vi "All Rounds.vi"(1 "Hash Function in":refnum<class "NI_SHA-3.lvclass">) -> (0 "Hash Function out":refnum<class "NI_SHA-3.lvclass">)   [LabVIEW 2020, in "NI_SHA-3.lvclass"]
uses:
  <vilib>/security/Message Digest/SHA-3/NI_SHA-3.lvclass
  <vilib>/security/Message Digest/SHA-3/NI_SHA-3.lvclass/NI_SHA-3.ctl
  a6197f31-9067-4d7d-80c5-9a64d9879faa.vi
  a6197f31-9067-4d7d-80c5-9a64d9879faa.vi/a07fe380-13ad-3f96-aad6-c8c87e91e43f.vi
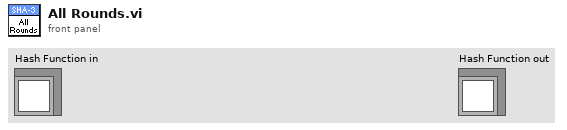
[diagram p1: front panel]
types:
  T1 = typedef "NI_SHA-3.lvclass/state.ctl" = cluster{"A00":T2, "A01":T2, "A02":T2, "A03":T2, "A04":T2, "A05":T2, "A06":T2, "A07":T2, "A08":T2, "A09":T2, "A10":T2, "A11":T2, "A12":T2, "A13":T2, "A14":T2, "A15":T2, "A16":T2, "A17":T2, "A18":T2, "A19":T2, "A20":T2, "A21":T2, "A22":T2, "A23":T2, "A24":T2}
  T2 = typedef "NI_SHA-3.lvclass/state word.ctl" = u64
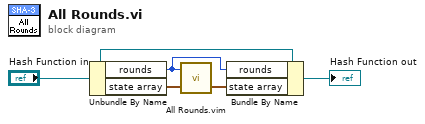
[diagram p0: block diagram]
diagram:
  n1 = Unbundle By Name("Hash Function in") -> ("rounds"=w3:i32, "state array"=w1:T1)
  n2 = call "All Rounds.vim"("state in"=w1, "rounds"=w3) -> ("state out"=w2:T1)  [unwired: 1 in]
  n3 = Bundle By Name(cluster="Hash Function in", "rounds"=w3, "state array"=w2) -> (→"Hash Function out":refnum<class "NI_SHA-3.lvclass">)
